vi "RichToFlatrfcontrol_CustomRequest.vi"(5 "OutputClusterType":T1, 11 "InputCluster":T2) -> (3 "OutputCluster":T1)   [LabVIEW 2024, in "FlexSDR_gRPC_client.lvlib"]
uses:
  FlexSDR_gRPC_client.lvlib
  rfcontrol_CustomRequest.ctl
  rfcontrol_CustomRequest_Flat.ctl
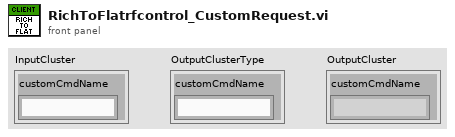
[diagram p1: front panel]
types:
  T1 = typedef "FlexSDR_gRPC_client.lvlib/rfcontrol_CustomRequest_Flat.ctl" = cluster{"customCmdName":string}
  T2 = typedef "FlexSDR_gRPC_client.lvlib/rfcontrol_CustomRequest.ctl" = cluster{"customCmdName":string}
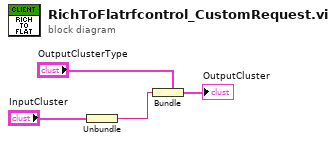
[diagram p0: block diagram]
diagram:
  n1 = Unbundle "Unbundle"("InputCluster") -> ("customCmdName"=w1:string)
  n2 = Bundle "Bundle"(cluster="OutputClusterType", "customCmdName"=w1) -> (→"OutputCluster":T1)
